vi "AttachDataSocket.vi"(7 "Enabled":bool, 8 "error in (no error)":errorcluster, 9 "Mode":T1(ring), 10 "URL":string, 11 "Control in":refnum<class "Control.lvclass">) -> (0 "error out":errorcluster, 3 "Control out":refnum<class "Control.lvclass">)   [LabVIEW 2015, in "Control.lvclass"]
doc: "National Instruments recommends using front panel data binding through the Shared Variable Engine or using the Bind To Network Path method to attach a data connection to a control.\n\n\nThis method allows you to attach an opc, ftp, and http connection to a control on Windows, and a dstp and file connection to a control on all LabVIEW-supported platforms. You can add new connections only at edit time.\n\n This method is similar to the <b>Data Binding Selection</b>, <b>Path</b>, and <b>Access Type</b> options on the <b>Data Binding</b> page of the Properties dialog box.\n\n\n<b>Note</b> If you use this method with a Boolean control in a radio buttons control, this method returns an error.\n\nQControl Class wrapper around the <b>Control : Attach DataSocket Method</b>.\n<b> </b> <b> </b>\n©2016 Q Software Innovations, LLC (QSI)\nwritten by Quentin Alldredge\nproduced in LabVIEW 2015\n\nsupport@qsoftwareinnovations.com\nwww.qsoftwareinnovations.com\n\nAll rights reserved.\n\nRedistribution and use in source and binary forms, with or without modification, are permitted provided that the following conditions are met:\n\n * Redistributions of source code must retain the above copyright notice, this list of conditions and the following disclaimer.\n * Redistributions in binary form must reproduce the above copyright notice, this list of conditions and the following disclaimer in the documentation and/or other materials provided with the distribution.\n * Neither the name of Q Software Innovations, LLC. nor the names of its contributors may be used to endorse or promote products derived from this software without specific prior written permission.\n\nTHIS SOFTWARE IS PROVIDED BY THE COPYRIGHT HOLDERS AND CONTRIBUTORS \"AS IS\" AND ANY EXPRESS OR IMPLIED WARRANTIES, INCLUDING, BUT NOT LIMITED TO, THE IMPLIED WARRANTIES OF MERCHANTABILITY AND FITNESS FOR A PARTICULAR PURPOSE ARE DISCLAIMED. IN NO EVENT SHALL THE COPYRIGHT OWNER OR CONTRIBUTORS BE LIABLE FOR ANY DIRECT, INDIRECT, INCIDENTAL, SPECIAL, EXEMPLARY, OR CONSEQUENTIAL DAMAGES (INCLUDING, BUT NOT LIMITED TO, PROCUREMENT OF SUBSTITUTE GOODS OR SERVICES; LOSS OF USE, DATA, OR PROFITS; OR BUSINESS INTERRUPTION) HOWEVER CAUSED AND ON ANY THEORY OF LIABILITY, WHETHER IN CONTRACT, STRICT LIABILITY, OR TORT (INCLUDING NEGLIGENCE OR OTHERWISE) ARISING IN ANY WAY OUT OF THE USE OF THIS SOFTWARE, EVEN IF ADVISED OF THE POSSIBILITY OF SUCH DAMAGE."
uses:
  Control.lvclass
  Control.lvclass/Control.ctl
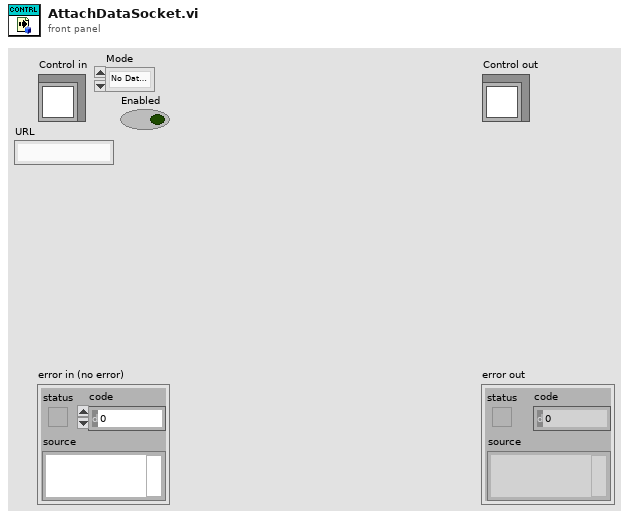
[diagram p1: front panel]
types:
  T1 = enum32{"No DataSocket", "Publish", "Subscribe", "Publish & Subscribe"}
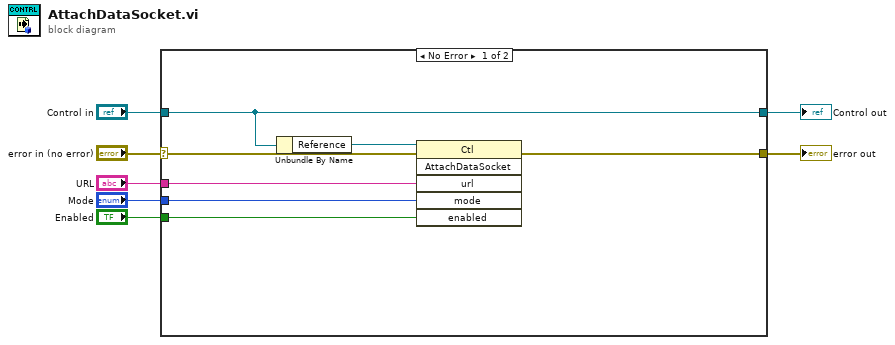
[diagram p0: block diagram]
diagram:
  n1 = case shown="No Error" "error in (no error)" {
    selector: "error in (no error)" -> [w14 w16]
    tunnel: [w13 w16] -> w6
    tunnel: [w12 w15] -> w4
    tunnel: "Control in" -> [w12 w15]
    tunnel: "URL" -> [w10 _]
    tunnel: "Mode" -> [w9 _]
    tunnel: "Enabled" -> [w8 _]
    frame No Error {
      n2 = Unbundle By Name(w12) -> ("Reference"=w11:refnum<vi>)
      n3 = invoke class="Ctl" method="AttachDataSocket"(reference=w11, error in=w14, "url"=w10, "mode"=w9, "enabled"=w8) -> (error out=w13:errorcluster)  [unwired: 1 in, 5 out]
    }
    frame Error {
    }
  }
  "error out" <- w6
  "Control out" <- w4
